vi "Power_Signal.vi"(9 "power signal frequency":dbl=10.0 format="%0.2p", 10 "Sampling Info":T1={"rate"=1000.0, "samples per channel"=1000} {"rate" format="%0.2f"}, 11 "physical channels":tag) -> ()   [LabVIEW 2014]
uses:
  Sampling_Info.ctl
  <vilib>/DAQmx/write.llb/DAQmx Write (Analog Wfm 1Chan NSamp).vi
  <vilib>/DAQmx/create/channels.llb/DAQmx Create Channel (AO-Voltage-Basic).vi
  <vilib>/DAQmx/miscellaneous.llb/DAQmx Fill In Error Info.vi
  <vilib>/measure/NI_MABase.lvlib
panel:
  in  "stop":bool
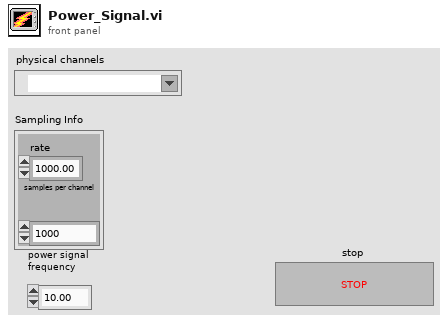
[diagram p1: front panel]
types:
  T1 = typedef "Sampling_Info.ctl" = cluster{"rate":dbl, "samples per channel":i32}
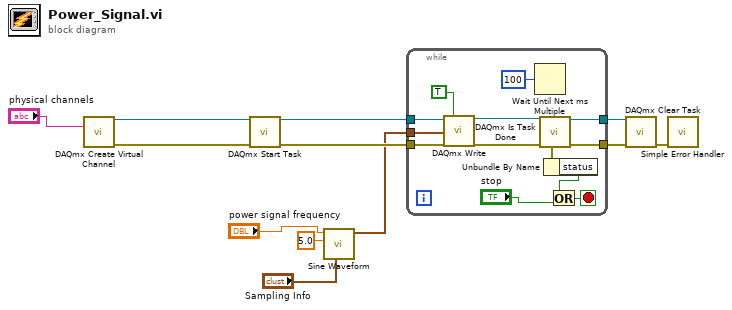
[diagram p0: block diagram]
diagram:
  n1 = call-poly <vilib>:"DAQmx Create Virtual Channel.vi"("physical channels"="physical channels") -> ("task out"=w7:refnum<k21>, "error out"=w6:errorcluster)  [unwired: 13 in]
  n2 = call <vilib>:"DAQmx Start Task.vi"("task/channels in"=w7, "error in"=w6) -> ("task out"=w3:refnum<k21>, "error out"=w2:errorcluster)  [unwired: 12 in]
  n3 = call <vilib>:"Sine Waveform.vi"("sampling info"="Sampling Info", "amplitude"=5.0, "frequency"="power signal frequency") -> ("signal out"=w1:waveform(dbl))  [unwired: 7 in, 1 out]
  n4 = while {
    tunnel: w3 -> [w14]
    tunnel: w2 -> [w23]
    tunnel: [w19] -> w10
    tunnel: [w22] -> w9
    tunnel: w1 -> [w16]
    stop <- w21 stop-if-true
    n5 = call-poly <vilib>:"DAQmx Write.vi"("task/channels in"=w14, "auto start"=TRUE, "data"=w16) -> ("task out"=w13:refnum<k21>)  [unwired: 10 in, 2 out]
    n6 = Wait Until Next ms Multiple(millisecond multiple=u32 100) -> ()  [unwired: 1 out]
    n7 = call <vilib>:"DAQmx Is Task Done.vi"("task/channels in"=w13, "error in"=w23) -> ("task out"=w22:refnum<k21>, "error out"=w19:errorcluster)  [unwired: 11 in, 1 out]
    n8 = Unbundle By Name(w19) -> ("status"=w18:bool)
    n9 = Or(x=w18, y="stop") -> (x .or. y?=w21:bool)
  }
  n10 = call <vilib>:"DAQmx Clear Task.vi"("task in"=w9, "error in"=w10) -> ("error out"=w11:errorcluster)  [unwired: 13 in]
  n11 = call <vilib>:"Simple Error Handler.vi"("error in (no error)"=w11) -> ()  [unwired: 4 in, 5 out]
